vi "PCI1220U角度置零.vi"(11 "AxisHandle IN":u32) -> (3 "AxisHandle OUT":u32)   [LabVIEW 2013]
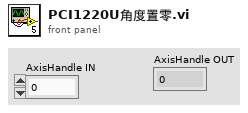
[diagram p1: front panel]
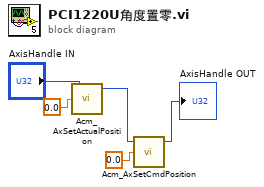
[diagram p0: block diagram]
diagram:
  n1 = call <userlib>:"Acm_AxSetActualPosition.vi"("Position"=0.0, "AxisHandle"="AxisHandle IN") -> ("AxisHandle"=w2:u32)  [unwired: 1 in, 2 out]
  n2 = call <userlib>:"Acm_AxSetCmdPosition.vi"("Position"=0.0, "AxisHandle"=w2) -> ("AxisHandle"=→"AxisHandle OUT":u32)  [unwired: 1 in, 2 out]
